vi "Remove Comments.vi"(8 "Error In":errorcluster, 11 "Original Settings File Contents":string) -> (0 "Error Out":errorcluster, 3 "Temp Settings File Contents (comments removed)":string)   [LabVIEW 2016, in "Error Manager.lvlib" / "Settings.lvclass"]
doc: "This VI opens the temporary copy of the Error Manager settings file, and alters the copy file by removing any comments from that file.\n\nComments are strings that start with the hashtag (#) character."
uses:
  Settings.lvclass
  OpenG VIs/OpenG VIs.lvclass
  <vilib>/Utility/error.llb/whitespace.ctl
panel:
  # "Development\nControls or indicators that are useful for development or testing, but which are not outputs of the VI."
  # "Input\nInputs to the VI"
  # "Output\nOutputs of the VI"
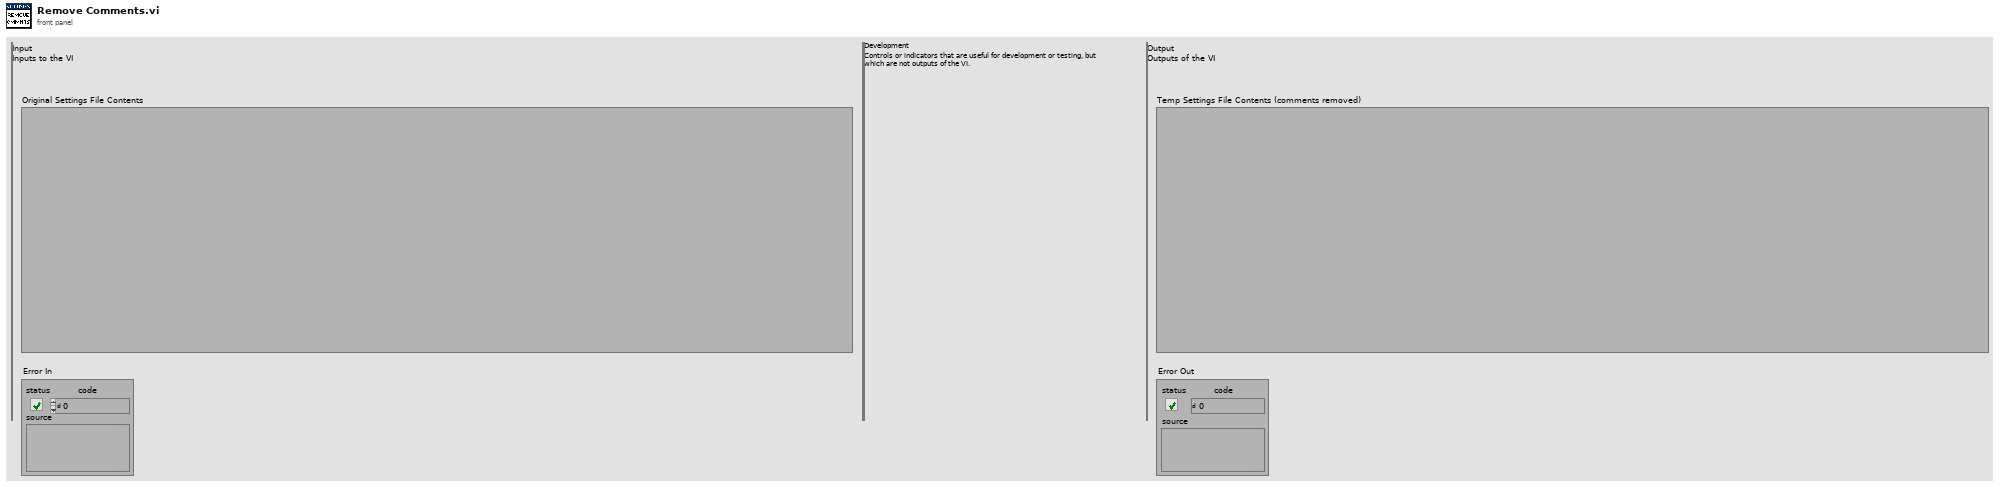
[diagram p1: front panel]
types:
  T1 = typedef "whitespace.ctl" = u16
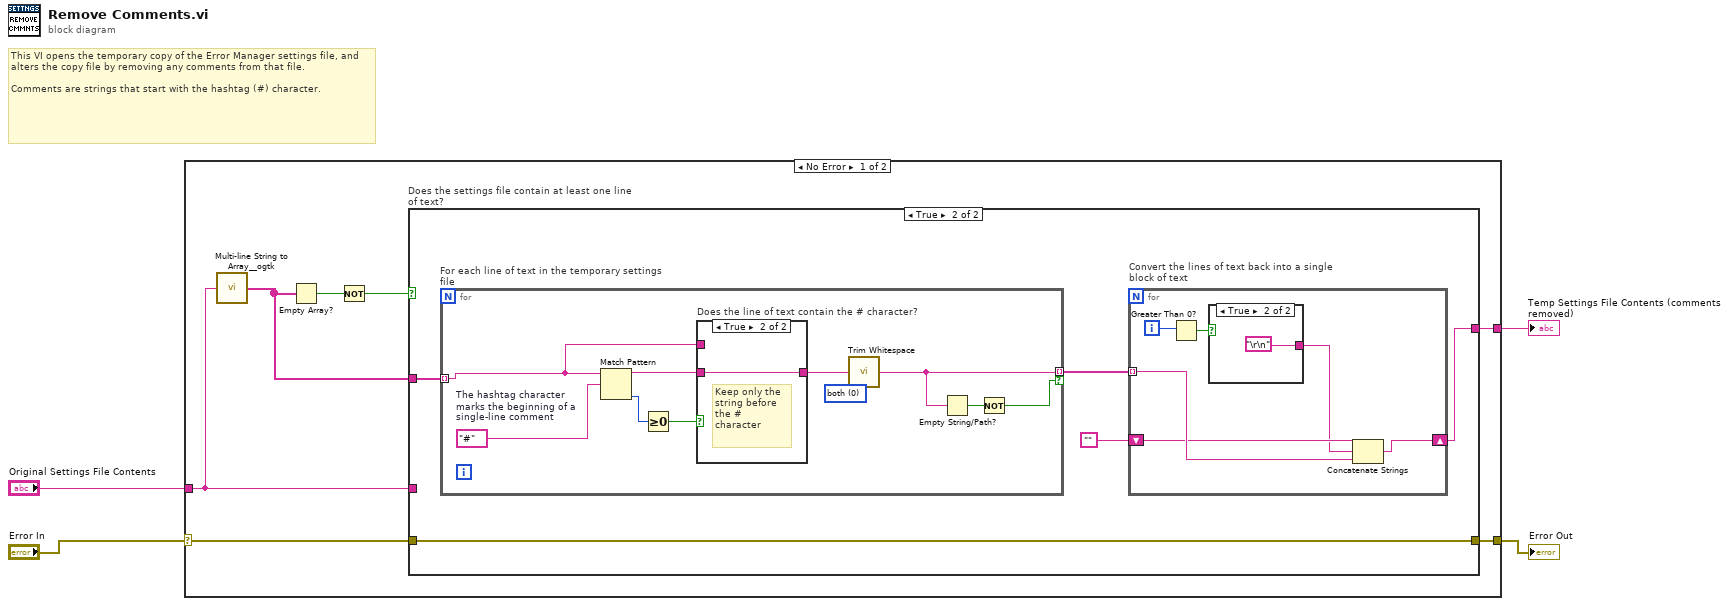
[diagram p0: block diagram]
diagram:
  # "This VI opens the temporary copy of the Error Manager settings file, and alters the copy file by removing any comments from that file.\n\nComments are strings that start with the hashtag (#) character."
  n1 = case shown="No Error" "Error In" {
    selector: "Error In" -> [w11 w39]
    tunnel: [w10 w39] -> w3
    tunnel: "Original Settings File Contents" -> [w5 w38]
    tunnel: [w6 w38] -> w1
    frame No Error {
      n2 = call "Multi-line String to Array__ogtk.vi"("string"=w5) -> ("lines"=w7:string[])
      n3 = Empty Array?(array=w7) -> (empty?=w9:bool)
      n4 = Not(x=w9) -> (.not. x?=w8:bool)
      n5 = case "Does the settings file contain at least one line of text?" shown="True" w8 {
        tunnel: [w13 w18] -> w10
        tunnel: w11 -> [w13 w18]
        tunnel: w7 -> [_ w17]
        tunnel: [w12 w14] -> w6
        tunnel: w5 -> [w12 _]
        frame False {
          # "The file is empty. There are no comments to remove."
        }
        frame True {
          n6 = for "For each line of text in the temporary settings file" {
            tunnel: w17 -> [w28] mode=indexing
            tunnel: [w27] -> w15 mode=indexing if=w29
            w26 = T1 0 items=["both", "start of string", "end of string"] ("location (both)")
            w35 = "#"  # The hashtag character marks the beginning of a single-line comment
            n7 = Match Pattern(string=w28, regular expression=w35) -> (before substring=w32:string, offset past match=w34:i32)  [unwired: 1 in, 2 out]
            n8 = Greater Or Equal To 0?(x=w34) -> (x >= 0?=w33:bool)
            n9 = case "Does the line of text contain the # character?" shown="True" w33 {
              tunnel: w32 -> [_ w37]
              tunnel: [w36 w37] -> w31
              tunnel: w28 -> [w36 _]
              frame False {
                # "Keep the line of text as is"
              }
              frame True {
                # "Keep only the string before the # character"
              }
            }
            n10 = call <vilib>:"Trim Whitespace.vi"("string"=w31, "location (both)"=w26) -> ("trimmed string"=w27:string)
            n11 = Empty String/Path?(string/path=w27) -> (empty?=w30:bool)
            n12 = Not(x=w30) -> (.not. x?=w29:bool)
          }
          n13 = for "Convert the lines of text back into a single block of text" {
            shift-right: [w22] -> w14
            shift-left: "" -> [w23]
            tunnel: w15 -> [w24] mode=indexing
            i -> [w21]
            n14 = Greater Than 0?(x=w21) -> (x > 0?=w20:bool)
            n15 = case shown="True" w20 {
              tunnel: [_ "\r\n"] -> w19
              frame False {
              }
              frame True {
              }
            }
            n16 = Concatenate Strings(w23, w19, w24) -> (w22:string)
          }
        }
      }
    }
    frame Error {
    }
  }
  "Error Out" <- w3
  "Temp Settings File Contents (comments removed)" <- w1
